vi "solar_write LogPause.vi"(8 "error in (no error)":errorcluster, 10 "Pause":bool, 11 "solar in":refnum<class "solar.lvclass">) -> (0 "error out":errorcluster, 3 "solar out":refnum<class "solar.lvclass">)   [LabVIEW 2018, in "solar.lvclass"]
doc: "If true, this pauses the log listbox update. If false, this unpauses the log listbox updates. Note: The messages are still logged when the listbox display is paused."
uses:
  solar.lvclass
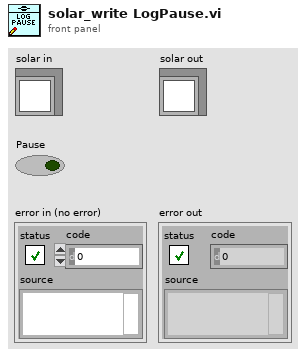
[diagram p1: front panel]
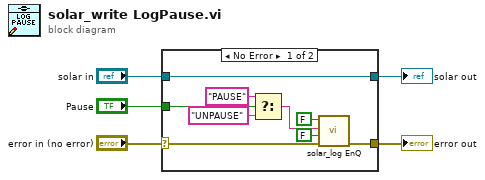
[diagram p0: block diagram]
diagram:
  n1 = case shown="No Error" "error in (no error)" {
    selector: "error in (no error)" -> [w13 w16]
    tunnel: "solar in" -> [w14 w15]
    tunnel: [w12 w16] -> w4
    tunnel: [w14 w15] -> w2
    tunnel: "Pause" -> [w9 _]
    frame No Error {
      n2 = Select(t="PAUSE" ("MSG"), s=w9, f="UNPAUSE" ("MSG")) -> (s? t:f=w6:string)
      n3 = call "solar_log EnQ.vi"("error in (no error)"=w13, "Front? (F)"=FALSE, "MSG"=w6, "Create? (F)"=FALSE) -> ("error out"=w12:errorcluster)  [unwired: 5 in, 2 out]
    }
    frame Error {
    }
  }
  "error out" <- w4
  "solar out" <- w2
